vi "ROI entry-Init ROI Entry globals.vi"(8 "error in (no error)":errorcluster) -> (0 "error out":errorcluster)   [LabVIEW 2013]
uses:
  ROI Entry screen/Typedefs/ROI input mode.ctl
  Visualisation/Functional Imaging Viewer/Typedefs/ROI parameters data type.ctl
  ROI Entry screen/Globals/gl_ROI Entry UI globals.vi
  Global Variables/General Globals.vi
  User profiles code/Globals/gl_UsrProfiles globals.vi
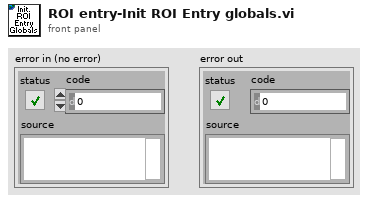
[diagram p1: front panel]
types:
  T1 = typedef "ROI parameters data type.ctl" = cluster{"ROI index":dbl, "ROI ID":dbl, "ROI Time (ns)":dbl, "Pixels in ROI":dbl, "X start":dbl, "Y start":dbl, "Z start":dbl, "X stop":dbl, "Y stop":dbl, "Z stop":dbl, "Angle (deg)":dbl, "Composite ID":dbl, "Number of lines":dbl, "Frame Size":dbl, "Zoom":dbl, "Laser Power (%)":dbl, "ROI group ID":dbl}
  T2 = typedef "ROI input mode.ctl" = enum16{"Unspecified", "Point-Line-Plane", "Volume"}
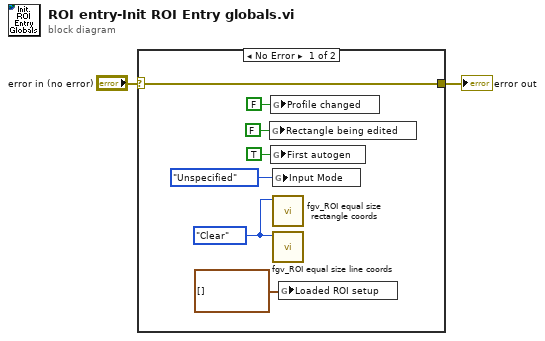
[diagram p0: block diagram]
diagram:
  n1 = case shown="No Error" "error in (no error)" {
    selector: "error in (no error)" -> [w6 w10]
    tunnel: [w6 w10] -> w2
    frame No Error {
      w5 = enum16{"Intialize", "Write", "Read", "Clear"}."Clear" ("Function")
      n2 = global write "gl_ROI Entry UI globals.vi" "Rectangle being edited"(FALSE ("Equal size is set")) -> ()
      n3 = global write "gl_UsrProfiles globals.vi" "Profile changed"(FALSE ("Profile changed")) -> ()
      n4 = global write "General Globals.vi" "First autogen"(TRUE ("First autogen")) -> ()
      n5 = global write "gl_ROI Entry UI globals.vi" "Input Mode"(ROI_input_mode."Unspecified" ("Input Mode")) -> ()
      n6 = call "fgv_ROI equal size rectangle coords.vi"("Function"=w5) -> ()  [unwired: 9 in, 2 out]
      n7 = call "fgv_ROI equal size line coords.vi"("Function"=w5) -> ()  [unwired: 9 in, 2 out]
      n8 = global write "gl_ROI Entry UI globals.vi" "Loaded ROI setup"(T1[] [] ("Loaded ROI setup")) -> ()
    }
    frame Error {
    }
  }
  "error out" <- w2
